vi "Create Test from Object.vi"(11 "Test":refnum<class>) -> (3 "Test":refnum<class "Executioner.lvclass">)   [LabVIEW 2020, in "Test Executive.lvlib" / "Executioner.lvclass"]
uses:
  <vilib>/gpm_packages/@cs/test-executive/Source/Test Executive/Executioner/Executioner.lvclass
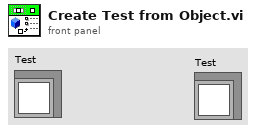
[diagram p1: front panel]
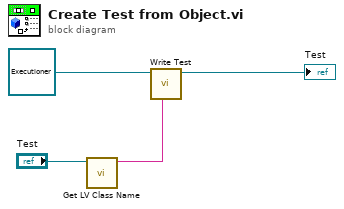
[diagram p0: block diagram]
diagram:
  n1 = call <vilib>:"Get LV Class Name.vi"("object"="Test") -> ("class name"=w2:string)  [unwired: 9 in, 1 out]
  n2 = call <vilib>:"Write Test.vi"("Test"=w2, "Executioner in"=refnum<class "Executioner.lvclass"> refnum ("Test")) -> ("Executioner out"=→"Test":refnum<class "Executioner.lvclass">)  [unwired: 9 in]
